vi "Traverse_Space_Server.vi"(6 "Probe Support":T1=[{"Max"=15.0, "Min"=-15.0}, {"Max"=250.0, "Min"=0.0}, {"Max"=15.0, "Min"=-15.0}] {"Min" format="%#.1f"; "Max" format="%#.1f"}, 7 "Mode":T4(ring), 8 "Traverse Limits":T1=[{"Max"=15001.0, "Min"=12000.0}, {"Max"=1000.0, "Min"=-1000.0}, {"Max"=700.0, "Min"=0.0}] {"Min" format="%#.1f"; "Max" format="%#.1f"}, 9 "Probe Volume":T1=[{"Max"=0.0, "Min"=0.0}, {"Max"=250.0, "Min"=0.0}, {"Max"=15.0, "Min"=-15.0}] {"Min" format="%#.1f"; "Max" format="%#.1f"}, 10 "Exclude Array":T2[](array[typedef]) {"Sizes"."Min" format="%#.1f"; "Sizes"."Max" format="%#.1f"}, 11 "Traverse Name":string) -> (0 "Traverse Limits Out":T1=[{"Max"=15001.0, "Min"=12000.0}, {"Max"=1000.0, "Min"=-1000.0}, {"Max"=700.0, "Min"=0.0}] {"Min" format="%#.1f"; "Max" format="%#.1f"}, 1 "Probe Volume Out":T1=[{"Max"=15.0, "Min"=-15.0}, {"Max"=250.0, "Min"=0.0}, {"Max"=15.0, "Min"=-15.0}] {"Min" format="%#.1f"; "Max" format="%#.1f"}, 2 "Exclude Array Out":T2[](array[typedef])=[{"Sizes"=[{"Max"=15000.0, "Min"=0.0}, {"Max"=1000.0, "Min"=-1000.0}, {"Max"=300.0, "Min"=0.0}], "Name"="Roughness Elements", "Exclude Type"=enum."Allow only vertical moves"}, {"Sizes"=[{"Max"=17000.0, "Min"=16000.0}, {"Max"=200.0, "Min"=-200.0}, {"Max"=-50.0, "Min"=-250.0}], "Name"="B204", "Exclude Type"=enum."Exclude completely"}] {"Sizes"."Min" format="%#.1f"; "Sizes"."Max" format="%#.1f"}, 3 "Error Comments":string, 4 "Probe Support Out":T1=[{"Max"=15.0, "Min"=-15.0}, {"Max"=250.0, "Min"=0.0}, {"Max"=15.0, "Min"=-15.0}] {"Min" format="%#.1f"; "Max" format="%#.1f"}, 5 "Space File":path)   [LabVIEW 2022 SP3]
uses:
  Gen Trav/Route mapping/Exclude_cluster.ctl
  Gen Trav/Route mapping/Box_size.ctl
  Gen Trav/Route mapping/Exclusion_type.ctl
  Globals/Constants_global.vi
  Globals/Trav_pos_global.vi
panel:
  # "(Relative to measurement position)"
  # "X                           Y                          Z"
  # "(Relative to measurement position)"
  # "X                           Y                          Z"
  # "X                           Y                          Z"
  # "X                           Y                          Z"
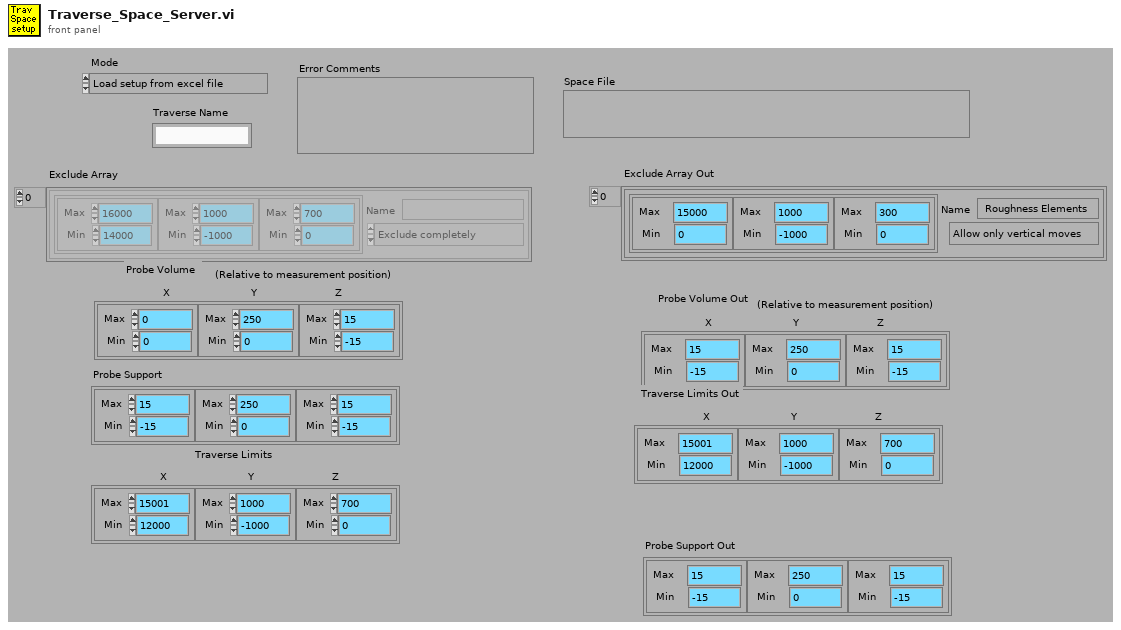
[diagram p1: front panel]
types:
  T1 = typedef "Box_size.ctl" = cluster{"Max":sgl, "Min":sgl}[]
  T2 = typedef "Exclude_cluster.ctl" = cluster{"Sizes":T1, "Name":string, "Exclude Type":T3}
  T3 = typedef "Exclusion_type.ctl" = enum16{"Exclude completely", "Allow only vertical moves"}
  T4 = enum16{"Load setup from excel file", "Save setup to excel file"}
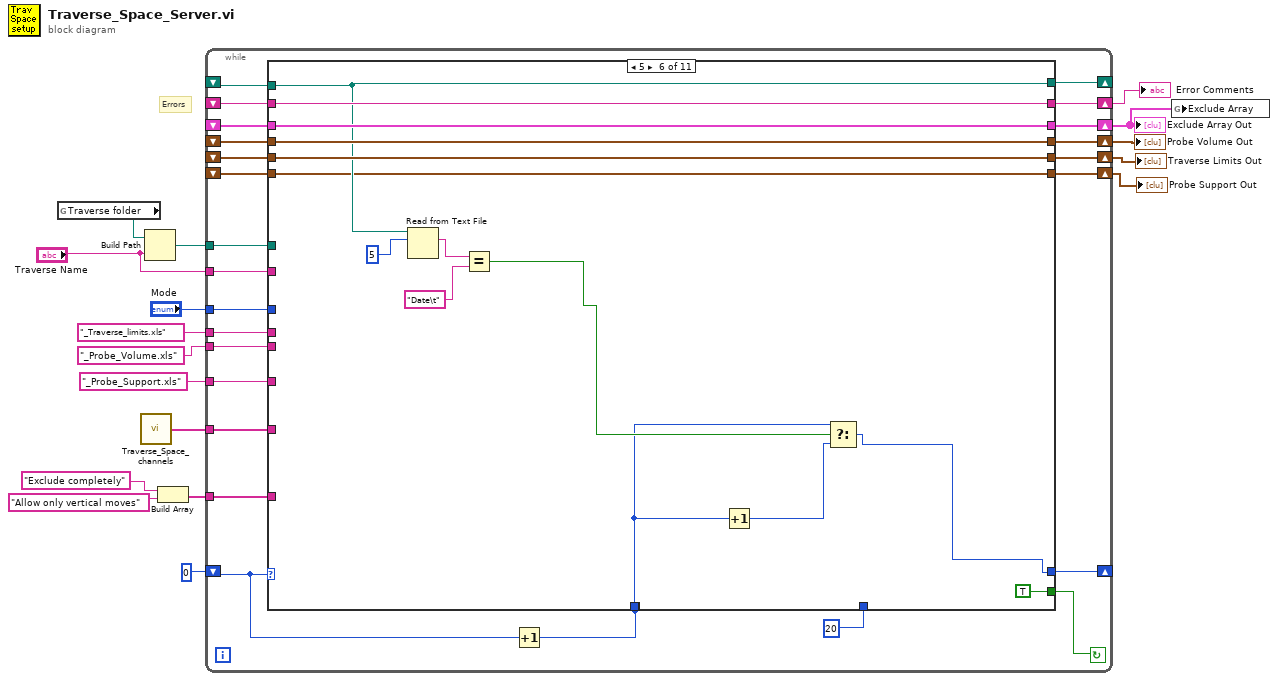
[diagram p0: block diagram]
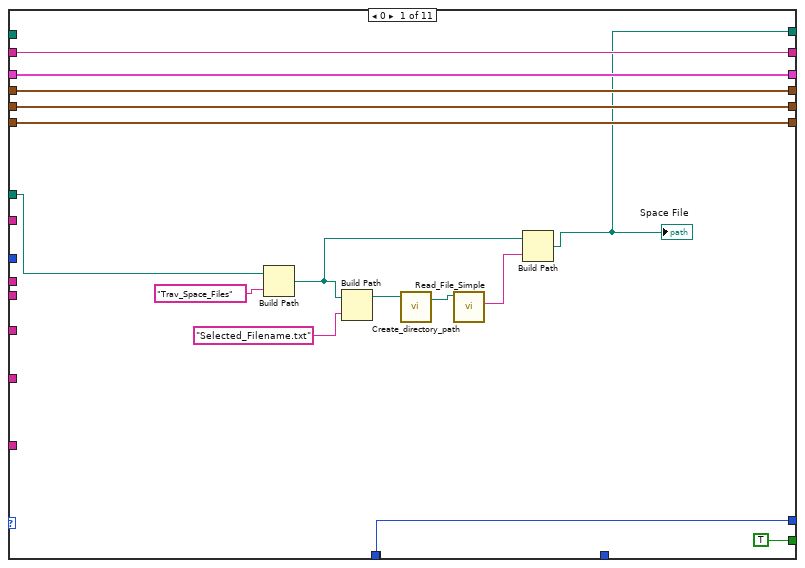
[diagram p2: hidden frame]
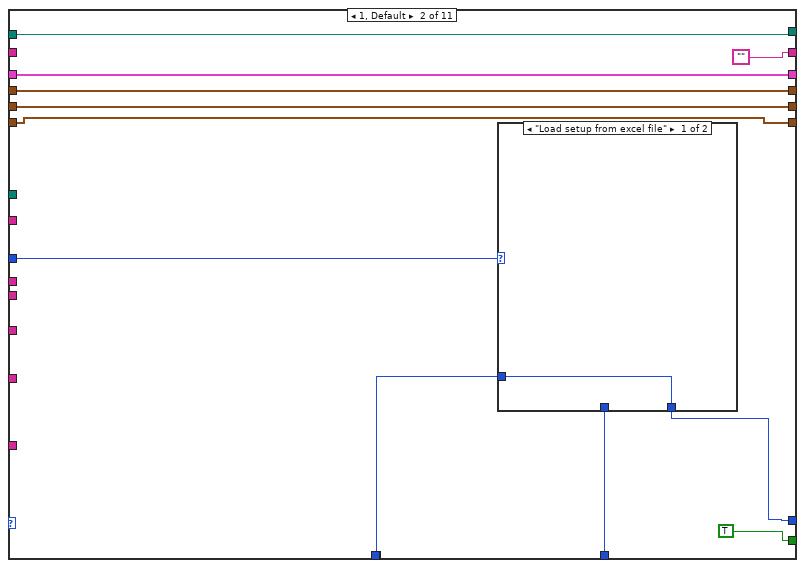
[diagram p3: hidden frame]
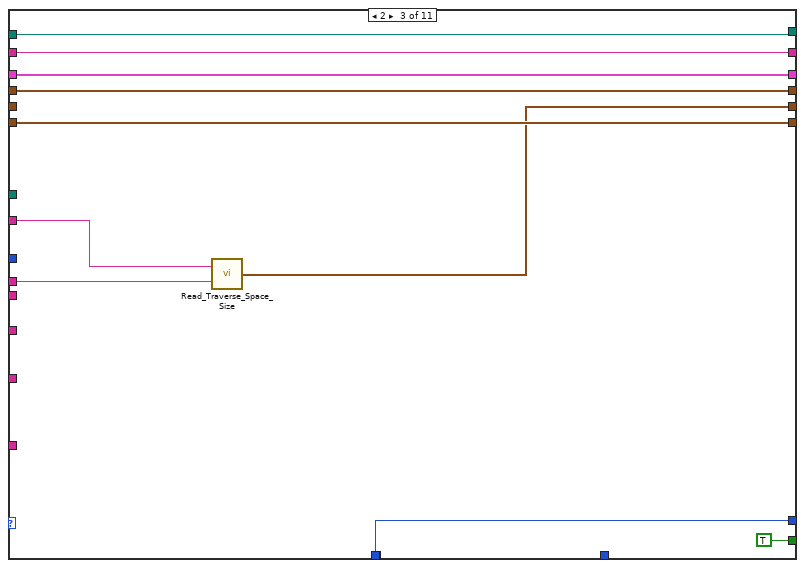
[diagram p5: hidden frame]
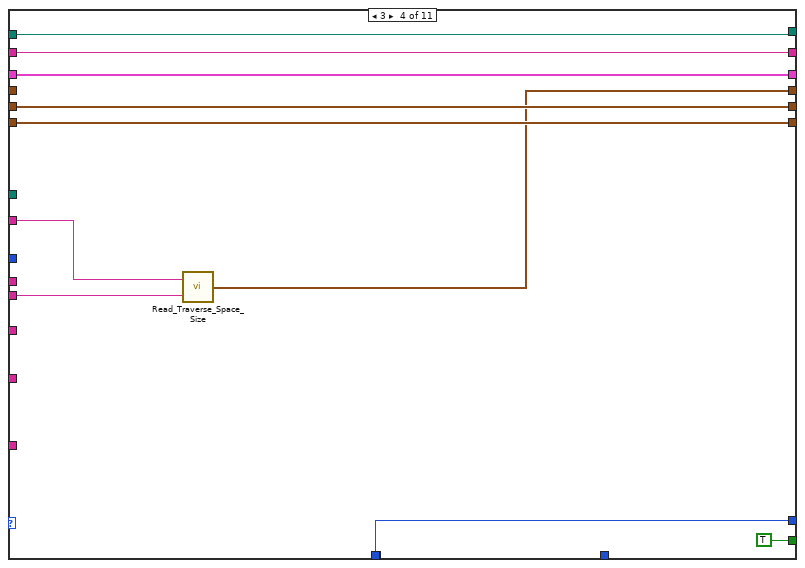
[diagram p6: hidden frame]
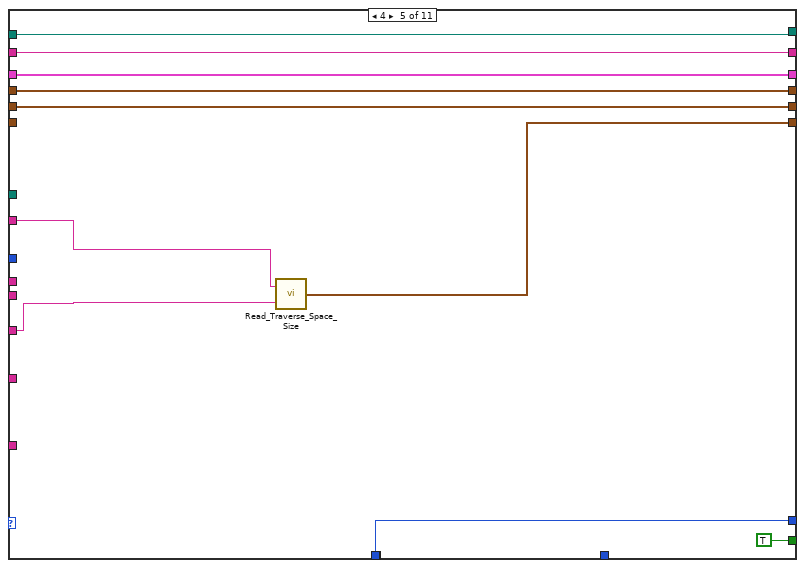
[diagram p7: hidden frame]
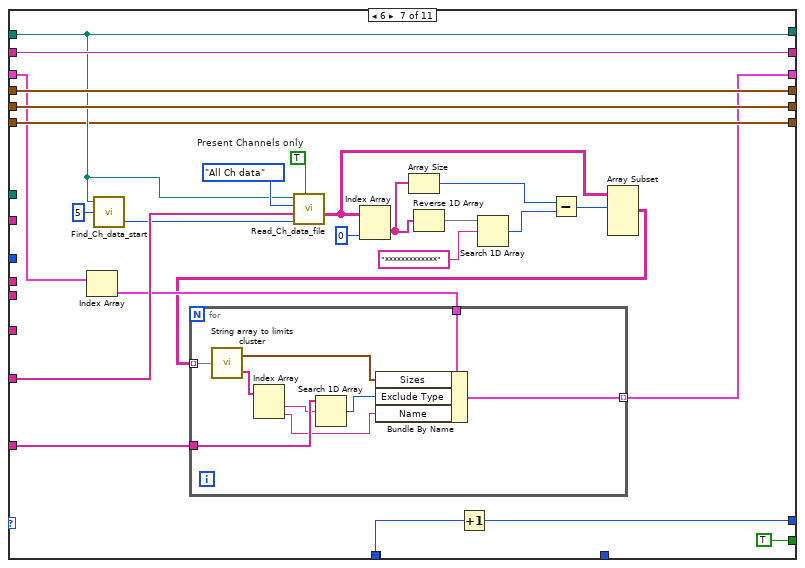
[diagram p8: hidden frame]
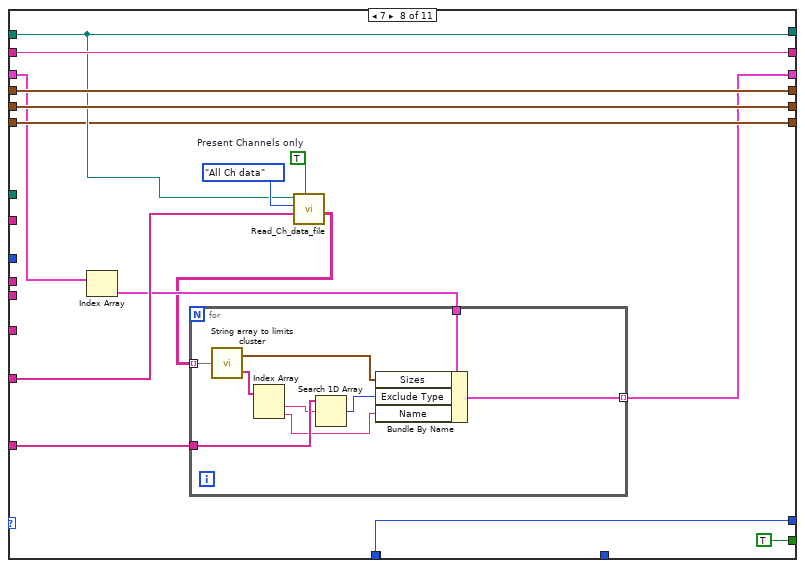
[diagram p9: hidden frame]
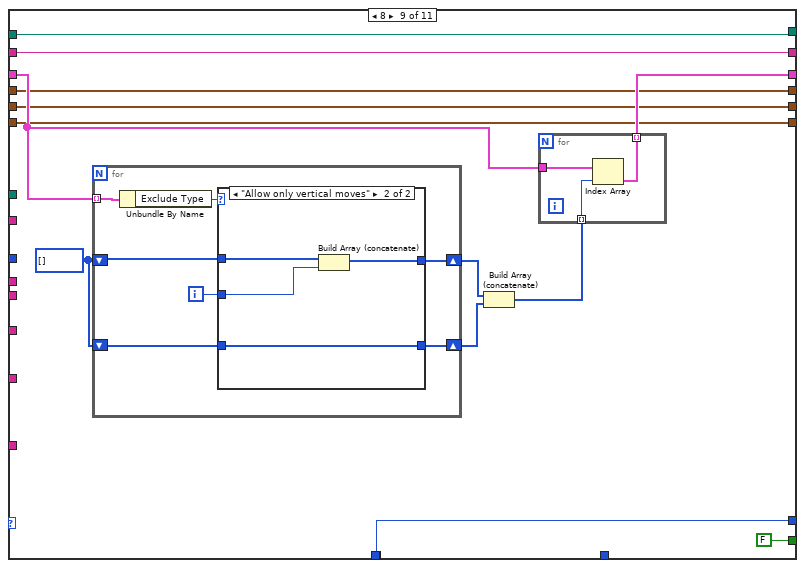
[diagram p10: hidden frame]
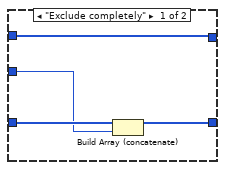
[diagram p11: hidden frame]
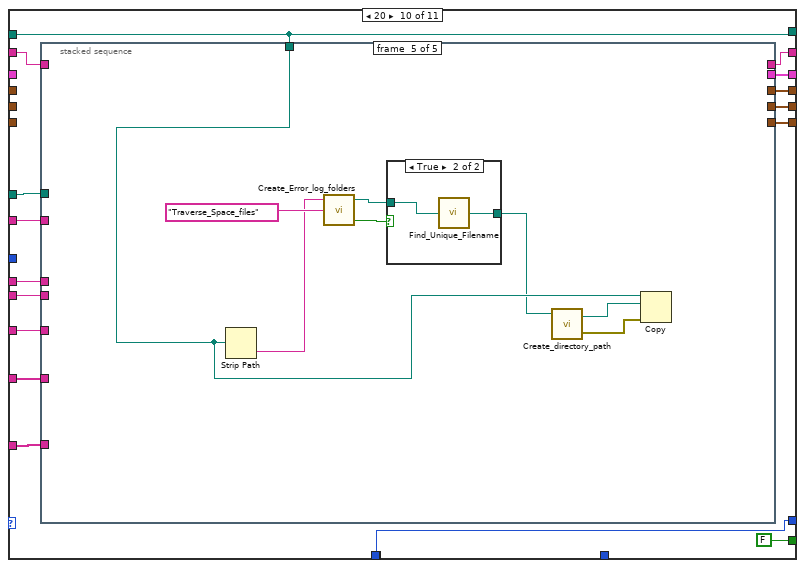
[diagram p12: hidden frame]
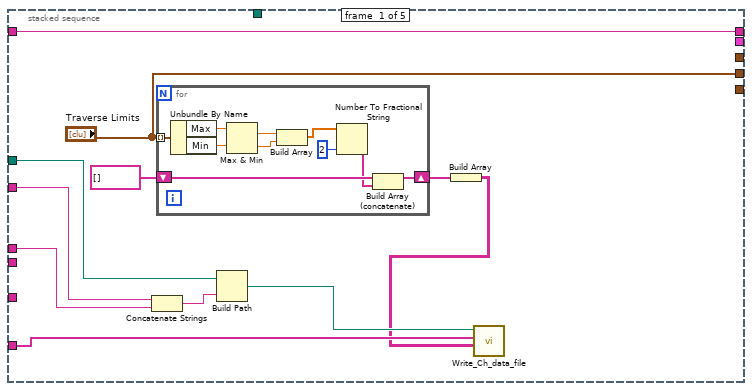
[diagram p13: hidden frame]
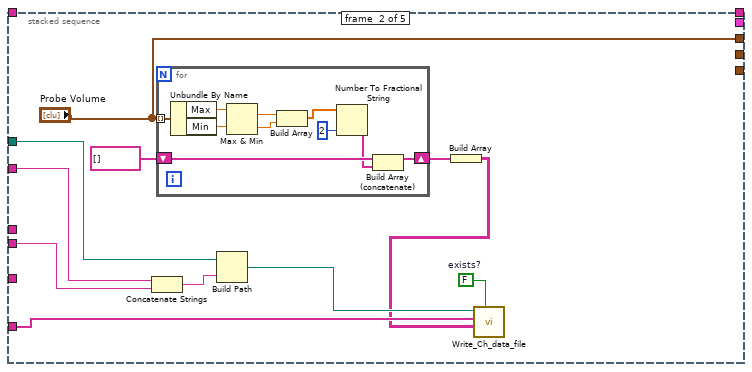
[diagram p14: hidden frame]
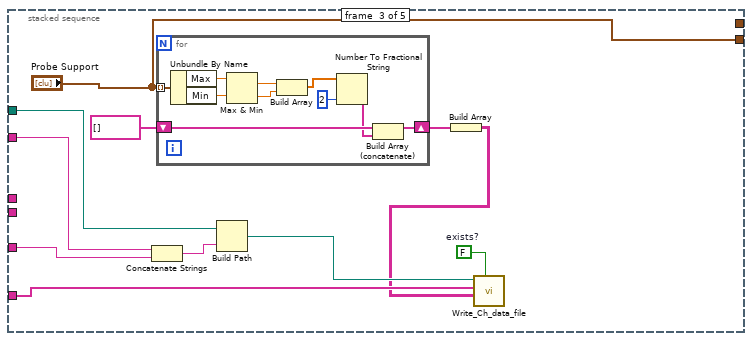
[diagram p15: hidden frame]
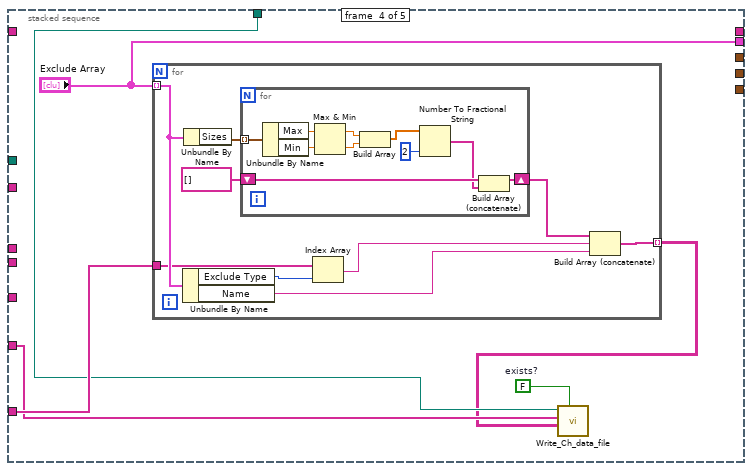
[diagram p16: hidden frame]
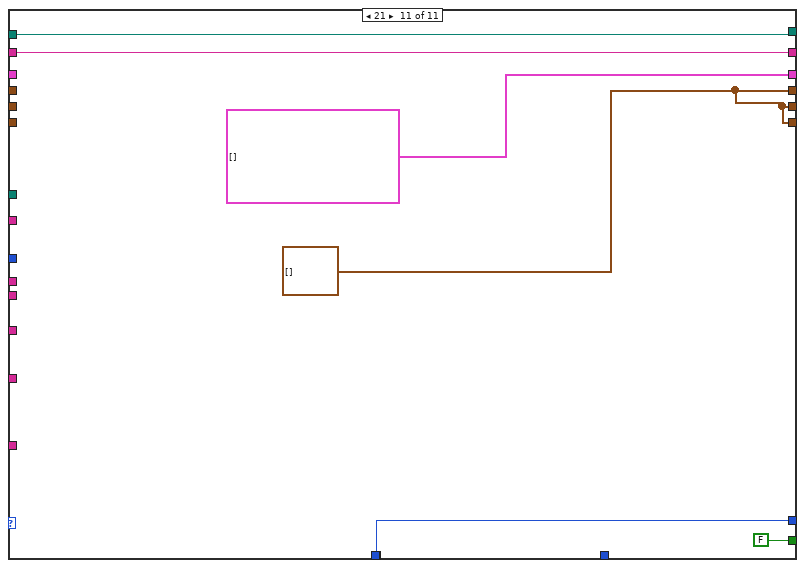
[diagram p18: hidden frame]
diagram:
  # "Errors"
  n1 = global read "Constants_global.vi" "Traverse folder"() -> (w7:path)
  n2 = call "Traverse_Space_channels.vi"() -> ("Channel Names"=w8:string[])
  n3 = Build Path(base path=w7, name or relative path="Traverse Name") -> (appended path=w6:path)
  n4 = Build Array("Exclude completely", "Allow only vertical moves") -> (w12:string[])
  n5 = while {
    tunnel: w12 -> [w29]
    shift-left: _ -> [w32]
    shift-right: [w31] -> w11
    tunnel: "Mode" -> [w39]
    shift-left: _ -> [w35]
    shift-right: [w34] -> w16
    shift-left: _ -> [w37]
    shift-right: [w36] -> w10
    shift-left: _ -> [w38]
    shift-right: [w28] -> w1
    shift-left: 0 -> [w41]
    shift-right: [w40] -> _
    shift-right: [w27] -> w9
    shift-left: _ -> [w26]
    shift-right: [w25] -> _
    shift-left: _ -> [w24]
    tunnel: w8 -> [w23]
    tunnel: w6 -> [w22]
    tunnel: "Traverse Name" -> [w21]
    tunnel: "_Traverse_limits.xls" ("string") -> [w20]
    tunnel: "_Probe_Volume.xls" ("string") -> [w19]
    tunnel: "_Probe_Support.xls" ("string") -> [w18]
    stop <- w42 continue-if-true
    n6 = Increment(x=w41) -> (x+1=w30:i32)
    n7 = case shown="5" w41 {
      tunnel: [TRUE TRUE TRUE TRUE TRUE TRUE TRUE TRUE FALSE FALSE FALSE] -> w42
      tunnel: w30 -> [w53 w64 _ _ _ _ _ _ w184 w213 w325]
      tunnel: [w53 w62 w76 w87 w98 w102 w115 w163 w184 w213 w325] -> w40
      tunnel: w39 -> [_ w68 _ _ _ _ _ _ _ _ _]
      tunnel: w38 -> [w56 w67 w75 w86 w97 w113 w117 w152 w179 _ _]
      tunnel: w37 -> [w55 w66 w80 _ w94 w110 w133 w157 w176 _ _]
      tunnel: [w55 w66 w80 w81 w94 w110 w133 w157 w176 w215 w321] -> w36
      tunnel: w35 -> [w54 w65 _ w84 w95 w111 w134 w158 w175 _ _]
      tunnel: [w54 w65 w71 w84 w95 w111 w134 w158 w175 w214 w321] -> w34
      tunnel: 20 -> [_ w63 _ _ _ _ _ _ _ _ _]
      tunnel: w32 -> [w57 _ w74 w85 w96 w112 w135 w159 w185 w217 w322]
      tunnel: [w57 "" w74 w85 w96 w112 w135 w159 w185 w218 w322] -> w31
      tunnel: w30 -> [_ _ w76 w87 w98 w104 w139 w163 _ _ _]
      tunnel: w29 -> [_ _ _ _ _ _ w120 w154 _ w219 _]
      tunnel: [w56 w67 w75 w86 w97 w113 w116 w151 w178 w216 T2[] [] ("Exclude Array")] -> w28
      tunnel: [w51 w61 w78 w89 w93 w101 w129 w155 w174 w212 w321] -> w27
      tunnel: w26 -> [w51 w61 w78 w89 _ w101 w129 w155 w174 _ _]
      tunnel: [w44 w60 w77 w88 w99 w109 w130 w156 w177 w211 w320] -> w25
      tunnel: w24 -> [_ w60 w77 w88 w99 w109 w130 w156 w177 w211 w320]
      tunnel: w23 -> [_ _ _ _ _ _ w136 w160 _ w207 _]
      tunnel: w22 -> [w43 _ _ _ _ _ _ _ _ w210 _]
      tunnel: w21 -> [_ _ w73 w83 w92 _ _ _ _ w209 _]
      tunnel: w20 -> [_ _ w72 _ _ _ _ _ _ w208 _]
      tunnel: w19 -> [_ _ _ w82 _ _ _ _ _ w206 _]
      tunnel: w18 -> [_ _ _ _ w91 _ _ _ _ w205 _]
      frame 0 {
        n8 = Build Path(base path=w43, name or relative path="Trav_Space_Files" ("Substring")) -> (appended path=w46:path)
        n9 = Build Path(base path=w46, name or relative path="Selected_Filename.txt" ("Substring")) -> (appended path=w50:path)
        n10 = call "Create_directory_path.vi"("Path name"=w50) -> ("Path name Out"=w49:path)  [unwired: 2 in, 1 out]
        n11 = call "Read_File_Simple.vi"("Filename"=w49) -> ("string"=w45:string)  [unwired: 2 in, 7 out]
        n12 = Build Path(base path=w46, name or relative path=w45) -> (appended path=w44:path)
        "Space File" <- w44
      }
      frame 1, Default {
        n13 = case shown="\"Load setup from excel file\"" w68 {
          tunnel: w64 -> [w69 _]
          tunnel: [w69 w70] -> w62
          tunnel: w63 -> [_ w70]
          frame "Load setup from excel file" {
          }
          frame "Save setup to excel file" {
          }
        }
      }
      frame 2 {
        n14 = call "Read_Traverse_Space_Size.vi"("Space_Name"=w72, "Traverse Name"=w73) -> ("Limits out"=w71:T1)
      }
      frame 3 {
        n15 = call "Read_Traverse_Space_Size.vi"("Space_Name"=w82, "Traverse Name"=w83) -> ("Limits out"=w81:T1)
      }
      frame 4 {
        n16 = call "Read_Traverse_Space_Size.vi"("Space_Name"=w91, "Traverse Name"=w92) -> ("Limits out"=w93:T1)
      }
      frame 5 {
        n17 = Read from Text File(file (use dialog)=w109, count=5) -> (text=w107:string)  [unwired: 2 in, 3 out]
        n18 = Equal?(x=w107, y="Date\t") -> (x = y?=w105:bool)
        n19 = Increment(x=w104) -> (x+1=w103:i32)
        n20 = Select(t=w104, s=w105, f=w103) -> (s? t:f=w102:i32)
      }
      frame 6 {
        w137 = TRUE  # Present Channels only
        n21 = Index Array(array=w117) -> (element=w119:T2)  [unwired: 1 in]
        n22 = call "Find_Ch_data_start.vi"("Approx No Of Columns"=5, "Filename"=w130) -> ("Start of read offset output"=w131:i32)  [unwired: 1 in, 2 out]
        n23 = call "Read_Ch_data_file.vi"("Present Channels only"=w137, "Start of read offset (chars.: 0)"=w131, "Present Channels"=w136, "Output"=enum16{"All Ch data", "The last few rows"}."All Ch data", "Filename"=w130) -> ("Channel Values"=w122:string[][])  [unwired: 4 out]
        n24 = Index Array(array=w122, index (col)=0 ("index (row)")) -> (element=w125:string[])  [unwired: 1 in]
        n25 = Array Size(array=w125) -> (size(s)=w124:i32)
        n26 = Reverse 1D Array(array=w125) -> (reversed array=w127:string[])
        n27 = Increment(x=w139) -> (x+1=w115:i32)
        n28 = Search 1D Array(1D array=w127, element="*************") -> (index of element=w123:i32)  [unwired: 1 in]
        n29 = Subtract(x=w124, y=w123) -> (x-y=w121:i32)
        n30 = Array Subset(array=w122, index (row)=w121) -> (w118:string[][])  [unwired: 3 in]
        n31 = for {
          tunnel: w120 -> [w148]
          tunnel: w119 -> [w146]
          tunnel: w118 -> [w142] mode=indexing
          tunnel: [w141] -> w116 mode=indexing
          n32 = call "String array to limits cluster.vi"("Channel Values in"=w142) -> ("Limits out"=w145:T1, "Channel Values out"=w149:string[])
          n33 = Index Array(array=w149) -> (element #1=w147:string, element #2=w144:string)  [unwired: 2 in]
          n34 = Search 1D Array(1D array=w148, element=w147) -> (index of element=w143:i32)  [unwired: 1 out]
          n35 = Bundle By Name(cluster=w146, "Sizes"=w145, "Exclude Type"=w143, "Name"=w144) -> (w141:T2)
        }
      }
      frame 7 {
        w161 = TRUE  # Present Channels only
        n36 = Index Array(array=w152) -> (element=w153:T2)  [unwired: 1 in]
        n37 = call "Read_Ch_data_file.vi"("Present Channels only"=w161, "Present Channels"=w160, "Output"=enum16{"All Ch data", "The last few rows"}."All Ch data", "Filename"=w156) -> ("Channel Values"=w150:string[][])  [unwired: 1 in, 4 out]
        n38 = for {
          tunnel: w154 -> [w172]
          tunnel: w153 -> [w170]
          tunnel: w150 -> [w166] mode=indexing
          tunnel: [w165] -> w151 mode=indexing
          n39 = call "String array to limits cluster.vi"("Channel Values in"=w166) -> ("Limits out"=w169:T1, "Channel Values out"=w173:string[])
          n40 = Index Array(array=w173) -> (element #1=w171:string, element #2=w168:string)  [unwired: 2 in]
          n41 = Search 1D Array(1D array=w172, element=w171) -> (index of element=w167:i32)  [unwired: 1 out]
          n42 = Bundle By Name(cluster=w170, "Sizes"=w169, "Exclude Type"=w167, "Name"=w168) -> (w165:T2)
        }
      }
      frame 8 {
        w183 = i32[] []
        n43 = for {
          tunnel: w179 -> [w190] mode=indexing
          shift-right: [w194] -> w181
          shift-left: w183 -> [w195]
          shift-right: [w193] -> w182
          shift-left: w183 -> [w192]
          i -> [w191]
          n44 = Unbundle By Name(w190) -> ("Exclude Type"=w196:T3)
          n45 = case shown="\"Allow only vertical moves\"" w196 {
            tunnel: w195 -> [w198 w204]
            tunnel: [w198 w203] -> w194
            tunnel: [w199 w202] -> w193
            tunnel: w192 -> [w200 w202]
            tunnel: w191 -> [w197 w201]
            frame "Exclude completely" {
              n46 = Build Array (concatenate)(w200, w197) -> (w199:i32[])
            }
            frame "Allow only vertical moves" {
              n47 = Build Array (concatenate)(w204, w201) -> (w203:i32[])
            }
          }
        }
        n48 = Build Array (concatenate)(w181, w182) -> (w180:i32[])
        n49 = for {
          tunnel: w180 -> [w189] mode=indexing
          tunnel: w179 -> [w188]
          tunnel: [w187] -> w178 mode=indexing
          n50 = Index Array(array=w188, index=w189) -> (element=w187:T2)
        }
      }
      frame 20 {
        n51 = stacked-sequence {
          tunnel: w219 -> [_ _ _ w289 _]
          tunnel: [w221 _ _ _ _] -> w218
          tunnel: w217 -> [w221 _ _ _ _]
          tunnel: [_ _ _ "Exclude Array" _] -> w216
          tunnel: [_ "Probe Volume" _ _ _] -> w215
          tunnel: ["Traverse Limits" _ _ _ _] -> w214
          tunnel: w211 -> [_ _ _ w287 w313]
          tunnel: [_ _ "Probe Support" _ _] -> w212
          tunnel: w210 -> [w229 w251 w272 _ _]
          tunnel: w209 -> [w228 w250 w271 _ _]
          tunnel: w208 -> [w226 _ _ _ _]
          tunnel: w207 -> [w224 w247 w268 w286 _]
          tunnel: w206 -> [_ w243 _ _ _]
          tunnel: w205 -> [_ _ w264 _ _]
          frame #0 {
            n52 = Concatenate Strings(w228, w226) -> (w227:string)
            n53 = for {
              shift-right: [w237] -> w223
              shift-left: string[] [] -> [w239]
              tunnel: "Traverse Limits" -> [w234] mode=indexing
              n54 = Unbundle By Name(w234) -> ("Max"=w233:sgl, "Min"=w232:sgl)
              n55 = Max & Min(x=w233, y=w232) -> (max(x,y)=w236:sgl, min(x,y)=w235:sgl)
              n56 = Build Array(w236, w235) -> (w241:sgl[])
              n57 = Number To Fractional String(number=w241, precision (6)=i16 2) -> (F-format string=w238:string[])  [unwired: 2 out]
              n58 = Build Array (concatenate)(w239, w238) -> (w237:string[])
            }
            n59 = Build Path(base path=w229, name or relative path=w227) -> (appended path=w225:path)
            n60 = Build Array(w223) -> (w222:string[][])
            n61 = call "Write_Ch_data_file.vi"("Channel Values"=w222, "Channel names"=w224, "Filename"=w225) -> ()  [unwired: 4 in, 5 out]
          }
          frame #1 {
            w242 = FALSE  # exists?
            n62 = Concatenate Strings(w250, w243) -> (w249:string)
            n63 = for {
              shift-right: [w258] -> w246
              shift-left: string[] [] -> [w260]
              tunnel: "Probe Volume" -> [w255] mode=indexing
              n64 = Unbundle By Name(w255) -> ("Max"=w254:sgl, "Min"=w253:sgl)
              n65 = Max & Min(x=w254, y=w253) -> (max(x,y)=w257:sgl, min(x,y)=w256:sgl)
              n66 = Build Array(w257, w256) -> (w262:sgl[])
              n67 = Number To Fractional String(number=w262, precision (6)=i16 2) -> (F-format string=w259:string[])  [unwired: 2 out]
              n68 = Build Array (concatenate)(w260, w259) -> (w258:string[])
            }
            n69 = Build Path(base path=w251, name or relative path=w249) -> (appended path=w248:path)
            n70 = Build Array(w246) -> (w245:string[][])
            n71 = call "Write_Ch_data_file.vi"("exists?"=w242, "Channel Values"=w245, "Channel names"=w247, "Filename"=w248) -> ()  [unwired: 3 in, 5 out]
          }
          frame #2 {
            w263 = FALSE  # exists?
            n72 = Concatenate Strings(w271, w264) -> (w270:string)
            n73 = for {
              shift-right: [w279] -> w267
              shift-left: string[] [] -> [w281]
              tunnel: "Probe Support" -> [w276] mode=indexing
              n74 = Unbundle By Name(w276) -> ("Max"=w275:sgl, "Min"=w274:sgl)
              n75 = Max & Min(x=w275, y=w274) -> (max(x,y)=w278:sgl, min(x,y)=w277:sgl)
              n76 = Build Array(w278, w277) -> (w283:sgl[])
              n77 = Number To Fractional String(number=w283, precision (6)=i16 2) -> (F-format string=w280:string[])  [unwired: 2 out]
              n78 = Build Array (concatenate)(w281, w280) -> (w279:string[])
            }
            n79 = Build Path(base path=w272, name or relative path=w270) -> (appended path=w269:path)
            n80 = Build Array(w267) -> (w266:string[][])
            n81 = call "Write_Ch_data_file.vi"("exists?"=w263, "Channel Values"=w266, "Channel names"=w268, "Filename"=w269) -> ()  [unwired: 3 in, 5 out]
          }
          frame #3 {
            w284 = FALSE  # exists?
            n82 = for {
              tunnel: "Exclude Array" -> [w296] mode=indexing
              tunnel: w289 -> [w294]
              tunnel: [w290] -> w285 mode=indexing
              n83 = Unbundle By Name(w296) -> ("Exclude Type"=w295:T3, "Name"=w291:string)
              n84 = Unbundle By Name(w296) -> ("Sizes"=w298:T1)
              n85 = for {
                tunnel: w298 -> [w308] mode=indexing
                shift-right: [w303] -> w293
                shift-left: string[] [] -> [w305]
                n86 = Unbundle By Name(w308) -> ("Max"=w302:sgl, "Min"=w301:sgl)
                n87 = Max & Min(x=w302, y=w301) -> (max(x,y)=w300:sgl, min(x,y)=w299:sgl)
                n88 = Build Array(w300, w299) -> (w307:sgl[])
                n89 = Number To Fractional String(number=w307, precision (6)=i16 2) -> (F-format string=w304:string[])  [unwired: 2 out]
                n90 = Build Array (concatenate)(w305, w304) -> (w303:string[])
              }
              n91 = Index Array(array=w294, index=w295) -> (element=w292:string)
              n92 = Build Array (concatenate)(w293, w292, w291) -> (w290:string[])
            }
            n93 = call "Write_Ch_data_file.vi"("exists?"=w284, "Channel Values"=w285, "Channel names"=w286, "Filename"=w287) -> ()  [unwired: 3 in, 5 out]
          }
          frame #4 {
            n94 = Strip Path(path=w313) -> (name=w312:string)  [unwired: 1 out]
            n95 = call "Create_Error_log_folders.vi"("Log Filename"=w312, "Log Folder"="Traverse_Space_files") -> ("Local Log File"=w314:path, "exists?"=w315:bool)  [unwired: 4 in]
            n96 = case shown="True" w315 {
              tunnel: [w317 w319] -> w311
              tunnel: w314 -> [w317 w318]
              frame False {
              }
              frame True {
                n97 = call "Find_Unique_Filename.vi"("Path In"=w318) -> ("Unique Path Out"=w319:path)  [unwired: 1 in, 1 out]
              }
            }
            n98 = call "Create_directory_path.vi"("Path name"=w311) -> ("error out"=w309:errorcluster, "Path name Out"=w310:path)  [unwired: 2 in]
            n99 = Copy(8:w309, 10:w310, 11:w313) -> ()  [unwired: 5 out]
          }
        }
      }
      frame 21 {
        w321 = T1 [] ("Probe Volume")
      }
    }
  }
  "Error Comments" <- w11
  "Probe Volume Out" <- w10
  "Traverse Limits Out" <- w16
  "Exclude Array Out" <- w1
  "Probe Support Out" <- w9
  n100 = global write "Trav_pos_global.vi" "Exclude Array"(w1) -> ()
